vi "Settrigger_input_connector_raw.vi"(8 "error in (no error)":errorcluster, 10 "Set_Val":i32, 11 "OneOfTemplate in":refnum<class "niswitch_grpc_RouteTriggerInputRequest_trigger_input_connector_enum.lvclass">) -> (0 "error out":errorcluster, 3 "OneOfTemplate out":refnum<class "niswitch_grpc_RouteTriggerInputRequest_trigger_input_connector_enum.lvclass">)   [LabVIEW 2021, in "NI Switch_client.lvlib" / "niswitch_grpc_RouteTriggerInputRequest_trigger_input_connector_enum.lvclass"]
uses:
  niswitch_grpc_RouteTriggerInputRequest_trigger_input_connector_enum.lvclass
  niswitch_grpc_RouteTriggerInputRequest_trigger_input_connector_enum.lvclass/niswitch_grpc_RouteTriggerInputRequest_trigger_input_connector_enum.ctl
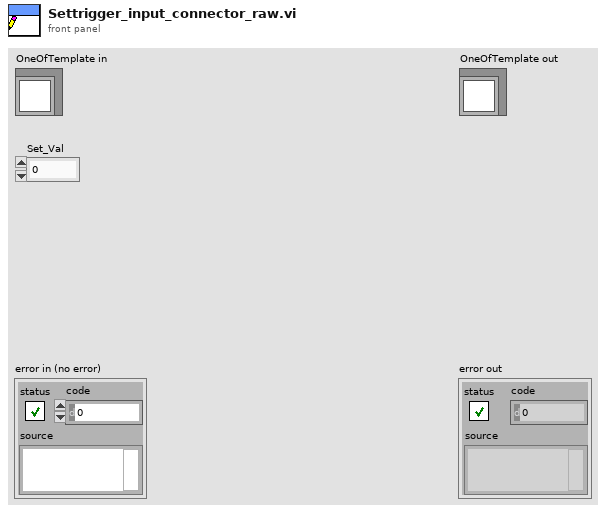
[diagram p1: front panel]
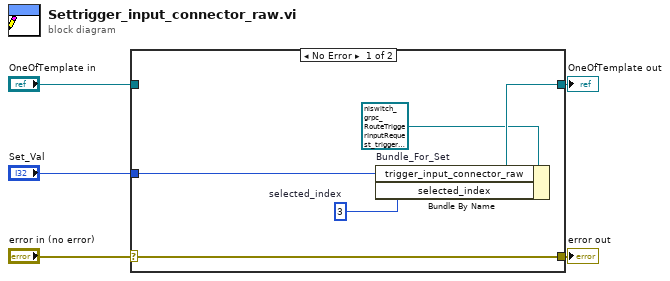
[diagram p0: block diagram]
diagram:
  n1 = case shown="No Error" "error in (no error)" {
    selector: "error in (no error)" -> [w10 w11]
    tunnel: [w10 w11] -> w4
    tunnel: [w9 w12] -> w2
    tunnel: "OneOfTemplate in" -> [_ w12]
    tunnel: "Set_Val" -> [w8 _]
    frame No Error {
      w7 = 3  # selected_index
      n2 = Bundle By Name "Bundle_For_Set"(cluster=refnum<class "niswitch_grpc_RouteTriggerInputRequest_trigger_input_connector_enum.lvclass"> refnum ("OneOfTemplate in"), "trigger_input_connector_raw"=w8, "selected_index"=w7) -> (w9:refnum<class "niswitch_grpc_RouteTriggerInputRequest_trigger_input_connector_enum.lvclass">)
    }
    frame Error {
    }
  }
  "error out" <- w4
  "OneOfTemplate out" <- w2
